vi "Run Banana Single Test.vi"() -> ()   [LabVIEW 2021]
uses:
  Banana.Caraya/Platano.CarayaTestSuite/Platano.CarayaTestSuite.lvclass
  Bananas/Bananas.lvlib
  Bananas/BananaPeel.Project/Project.lvclass
  Bananas/BananaPeel.Example/GUID.lvclass
  Bananas/Requirements/RequirementsMap.lvclass
  Bananas/AssertTrue/AssertTrue.lvclass
  C:/Repositories/LVOS/Bananas/lv-src/Bananas/BananaPeel/BananaPeel.lvclass
panel:
  out "Ephemeral Strategies":string[](array[string])
  in  "error in":errorcluster
  out "error out":errorcluster
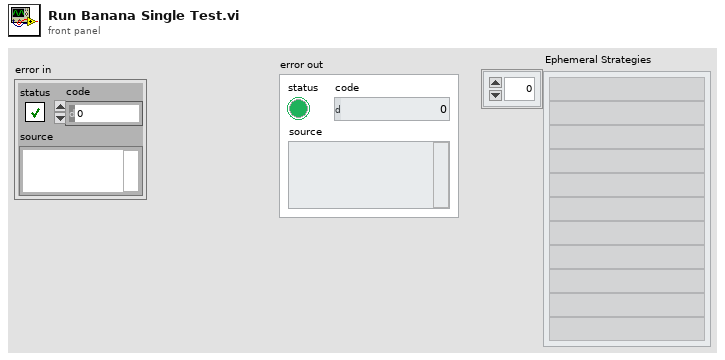
[diagram p1: front panel]
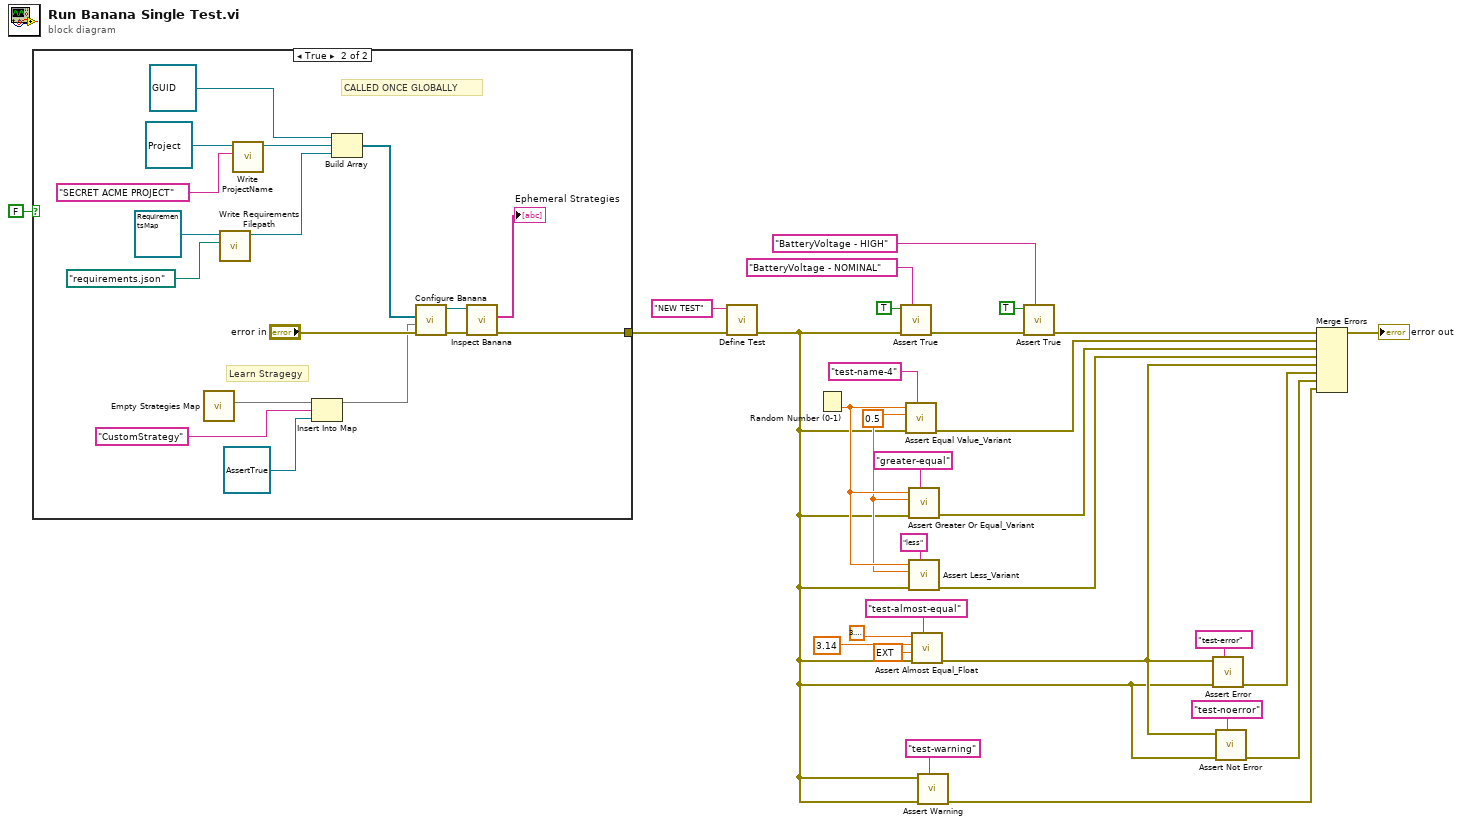
[diagram p0: block diagram]
diagram:
  w16 = 0.5
  n1 = case shown="True" FALSE {
    tunnel: [_ w36] -> w23
    frame False {
    }
    frame True {
      # "Learn Stragegy"
      # "CALLED ONCE GLOBALLY"
      n2 = call "Empty Strategies Map.vi"() -> ("Ephemeral Strategies"=w34:map{string, refnum<class "BananaPeel.lvclass">})  [unwired: 11 in]
      n3 = call "Write Requirements Filepath.vi"("File Path"=path "requirements.json", "Project in"=refnum<class "RequirementsMap.lvclass"> refnum ("Bananas.lvlib:RequirementsFile.lvclass")) -> ("Project out"=w40:refnum<class "RequirementsMap.lvclass">)  [unwired: 9 in]
      n4 = call "Write ProjectName.vi"("ProjectName"="SECRET ACME PROJECT" ("Label"), "Project in"=refnum<class "Project.lvclass"> refnum ("Bananas.lvlib:Project.lvclass")) -> ("Project out"=w43:refnum<class "Project.lvclass">)  [unwired: 9 in]
      n5 = Insert Into Map(map in=w34, key="CustomStrategy" ("Label"), value=refnum<class "AssertTrue.lvclass"> refnum ("Bananas.lvlib:AssertTrue.lvclass")) -> (map out=w33:map{string, refnum<class "BananaPeel.lvclass">})  [unwired: 2 out]
      n6 = Build Array(refnum<class "GUID.lvclass"> refnum ("Bananas.lvlib:Example.lvclass"), w43, w40) -> (w46:refnum<class "BananaPeel.lvclass">[])
      n7 = call "Configure Banana.vi"("error in"="error in", "Ephemeral Strategies"=w33, "Peels"=w46) -> ("error out"=w37:errorcluster, "Platano"=w38:refnum<class "Platano.lvclass">)  [unwired: 7 in]
      n8 = call "Inspect Banana.vi"("error in"=w37, "Platano"=w38) -> ("error out"=w36:errorcluster, "Ephemeral Strategies"=→"Ephemeral Strategies":string[])  [unwired: 7 in, 1 out]
    }
  }
  n9 = call "Define Test.vi"("error in"=w23, "Label (VI Title)"="NEW TEST") -> ("error out"=w3:errorcluster)  [unwired: 8 in, 1 out]
  n10 = Random Number (0-1)() -> (number: 0 to 1=w17:dbl)
  n11 = call "Assert True.vi"("Label"="BatteryVoltage - NOMINAL", "error in"=w3, "True?"=TRUE) -> ("error out"=w26:errorcluster)  [unwired: 7 in, 1 out]
  n12 = call "Assert Equal Value_Variant.vi"("Label"="test-name-4", "error in"=w3, "Y"=w16, "X"=w17) -> ("error out"=w21:errorcluster)  [unwired: 6 in, 1 out]
  n13 = call "Assert Greater Or Equal_Variant.vi"("Label"="greater-equal", "error in"=w3, "Y"=w16, "X"=w17) -> ("error out"=w19:errorcluster)  [unwired: 6 in, 1 out]
  n14 = call "Assert Less_Variant.vi"("Label"="less", "error in"=w3, "Y"=w16, "X"=w17) -> ("error out"=w14:errorcluster)  [unwired: 6 in, 1 out]
  n15 = call "Assert Almost Equal_Float.vi"("Label"="test-almost-equal", "error in"=w3, "Tolerance"=ext 0.00000100000000000000000004, "Y"=3.14, "X"=3.141592653589793) -> ("error out"=w4:errorcluster)  [unwired: 5 in, 1 out]
  n16 = call "Assert Warning.vi"("Label"="test-warning", "error in"=w3, "warning"=w3) -> ("error out"=w1:errorcluster)  [unwired: 7 in, 1 out]
  n17 = call "Assert True.vi"("Label"="BatteryVoltage - HIGH", "error in"=w26, "True?"=TRUE) -> ("error out"=w25:errorcluster)  [unwired: 7 in, 1 out]
  n18 = call "Assert Error.vi"("Label"="test-error", "error in"=w3, "error"=w4) -> ("error out"=w10:errorcluster)  [unwired: 7 in, 1 out]
  n19 = call "Assert Not Error.vi"("Label"="test-noerror", "error in"=w3, "error"=w4) -> ("error out"=w9:errorcluster)  [unwired: 7 in, 1 out]
  n20 = Merge Errors(w25, w21, w19, w14, w4, w10, w9, w1) -> (→"error out":errorcluster)
